vi "Check results (all plots).vi"(8 "error in":errorcluster, 9 "App Data":T1, 10 "XY Graph":refnum<vi>, 11 "ComboBox in":refnum<vi>) -> (0 "error out":errorcluster, 2 "results (short)":string, 3 "detailed results":string)   [LabVIEW 2014]
uses:
  Controls/App Data.ctl
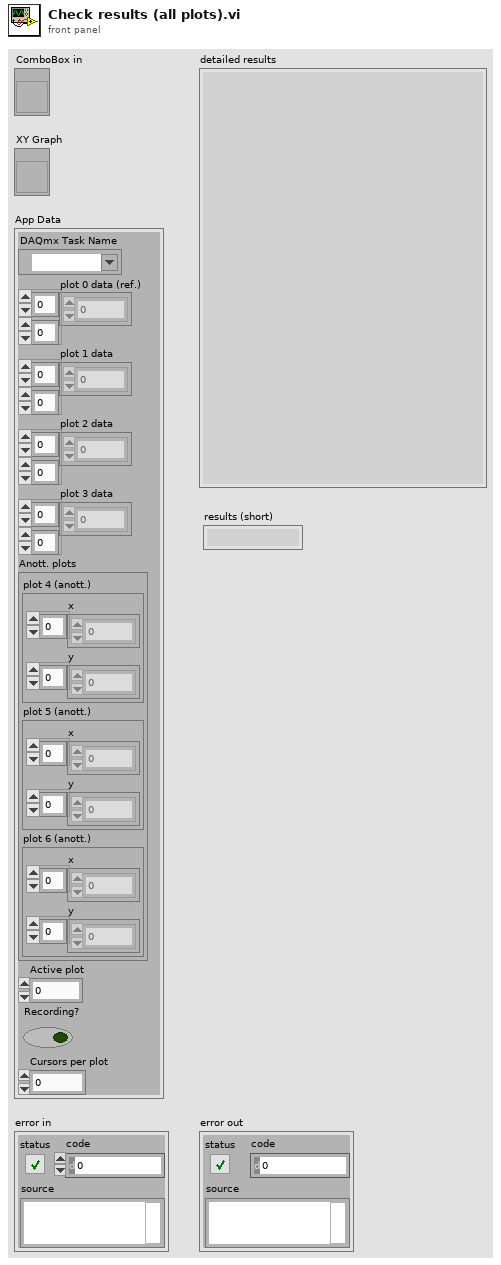
[diagram p1: front panel]
types:
  T1 = typedef "App Data.ctl" = cluster{"DAQmx Task Name":refnum<k21>, "plot 0 data (ref.)":dbl[][], "plot 1 data":dbl[][], "plot 2 data":dbl[][], "plot 3 data":dbl[][], "Anott. plots":cluster{"plot 4 (anott.)":cluster{"x":dbl[], "y":dbl[]}, "plot 5 (anott.)":cluster{"x":dbl[], "y":dbl[]}, "plot 6 (anott.)":cluster{"x":dbl[], "y":dbl[]}}, "Active plot":u32, "Recording?":bool, "Cursors per plot":i32}
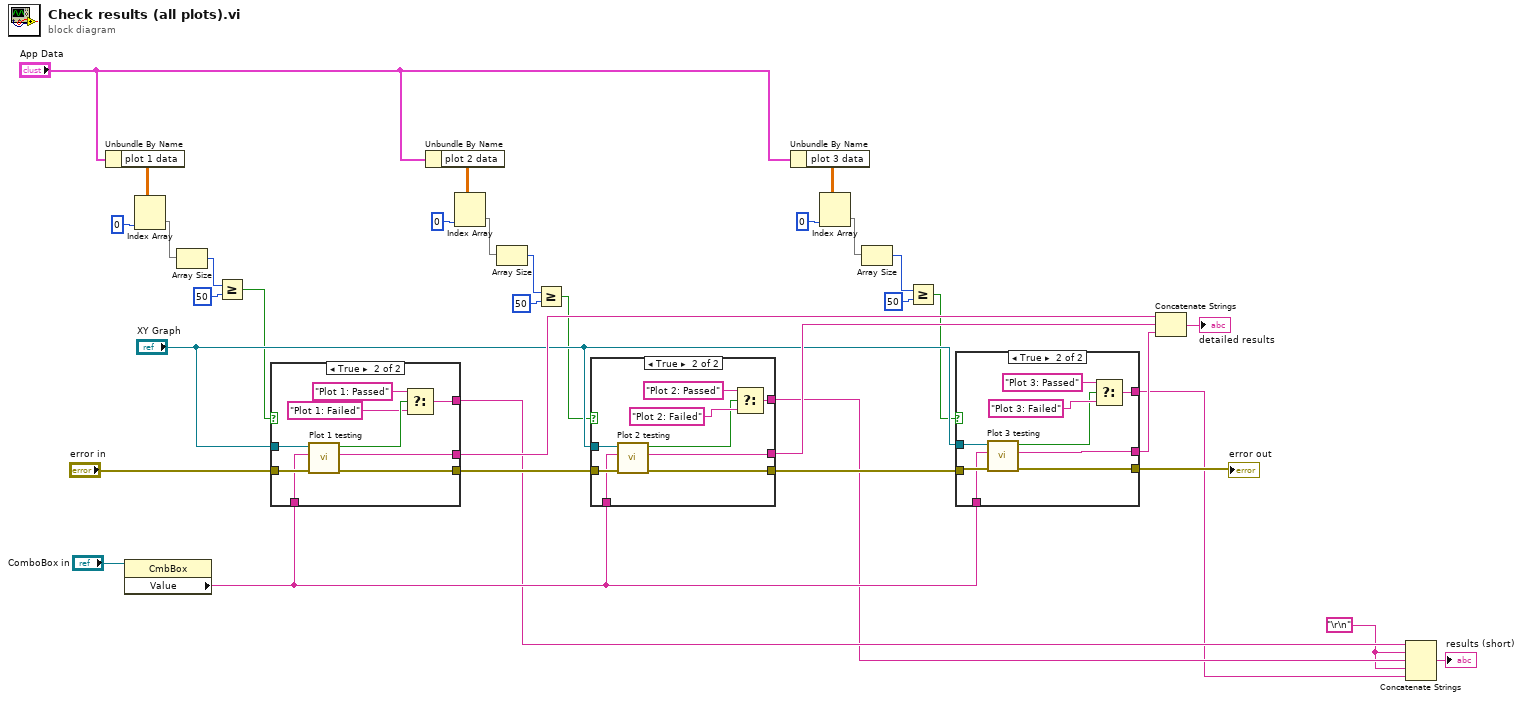
[diagram p0: block diagram]
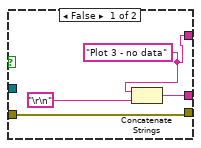
[diagram p2: hidden frame]
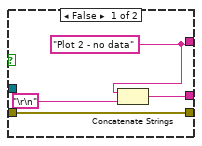
[diagram p3: hidden frame]
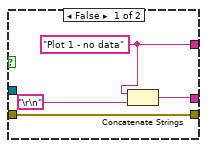
[diagram p4: hidden frame]
diagram:
  w3 = "\r\n"
  n1 = Unbundle By Name("App Data") -> ("plot 1 data"=w9:dbl[][])
  n2 = property class="CmbBox"(reference="ComboBox in") -> ("Value"=w31:string)  [unwired: 1 in, 2 out]
  n3 = Index Array(array=w9, index (col)=0 ("disabled index (col)")) -> (element=w10:dbl[])  [unwired: 1 in]
  n4 = Array Size(array=w10) -> (size(s)=w11:i32)
  n5 = Greater Or Equal?(x=w11, y=50) -> (x >= y?=w13:bool)
  n6 = case shown="True" w13 {
    tunnel: "error in" -> [w39 w48]
    tunnel: [w39 w47] -> w27
    tunnel: "XY Graph" -> [_ w46]
    tunnel: w31 -> [_ w45]
    tunnel: [w38 w44] -> w32
    tunnel: [w36 w40] -> w5
    frame False {
      w36 = "Plot 1 - no data" ("concatenated string 6")
      n7 = Concatenate Strings(w36, "\r\n") -> (w38:string)
    }
    frame True {
      n8 = call "Plot 1 testing.vi"("error in"=w48, "TWT type"=w45, "XY Graph"=w46) -> ("error out"=w47:errorcluster, "Results"=w44:string, "Plot 1 pass?"=w43:bool)  [unwired: 6 in]
      n9 = Select(t="Plot 1: Passed", s=w43, f="Plot 1: Failed") -> (s? t:f=w40:string)
    }
  }
  n10 = Unbundle By Name("App Data") -> ("plot 2 data"=w15:dbl[][])
  n11 = Index Array(array=w15, index (col)=0 ("disabled index (col)")) -> (element=w16:dbl[])  [unwired: 1 in]
  n12 = Array Size(array=w16) -> (size(s)=w17:i32)
  n13 = Greater Or Equal?(x=w17, y=50) -> (x >= y?=w19:bool)
  n14 = case shown="True" w19 {
    tunnel: w27 -> [w52 w61]
    tunnel: [w52 w60] -> w28
    tunnel: "XY Graph" -> [_ w59]
    tunnel: w31 -> [_ w58]
    tunnel: [w50 w57] -> w33
    tunnel: [w49 w53] -> w4
    frame False {
      w49 = "Plot 2 - no data" ("concatenated string 6")
      n15 = Concatenate Strings(w49, "\r\n") -> (w50:string)
    }
    frame True {
      n16 = call "Plot 2 testing.vi"("error in"=w61, "TWT type"=w58, "XY Graph"=w59) -> ("error out"=w60:errorcluster, "concatenated string 6"=w57:string, "Plot 2 pass?"=w54:bool)  [unwired: 6 in]
      n17 = Select(t="Plot 2: Passed", s=w54, f="Plot 2: Failed") -> (s? t:f=w53:string)
    }
  }
  n18 = Unbundle By Name("App Data") -> ("plot 3 data"=w21:dbl[][])
  n19 = Index Array(array=w21, index (col)=0 ("disabled index (col)")) -> (element=w22:dbl[])  [unwired: 1 in]
  n20 = Array Size(array=w22) -> (size(s)=w23:i32)
  n21 = Greater Or Equal?(x=w23, y=50) -> (x >= y?=w25:bool)
  n22 = case shown="True" w25 {
    tunnel: w28 -> [w65 w74]
    tunnel: [w65 w73] -> w29
    tunnel: "XY Graph" -> [_ w72]
    tunnel: w31 -> [_ w71]
    tunnel: [w63 w70] -> w34
    tunnel: [w62 w67] -> w2
    frame False {
      w62 = "Plot 3 - no data" ("concatenated string 6")
      n23 = Concatenate Strings(w62, "\r\n") -> (w63:string)
    }
    frame True {
      n24 = call "Plot 3 testing.vi"("error in"=w74, "TWT type"=w71, "XY Graph"=w72) -> ("error out"=w73:errorcluster, "concatenated string 6"=w70:string, "Plot 3 pass?"=w66:bool)  [unwired: 6 in]
      n25 = Select(t="Plot 3: Passed", s=w66, f="Plot 3: Failed") -> (s? t:f=w67:string)
    }
  }
  "error out" <- w29
  n26 = Concatenate Strings(w32, w33, w34) -> (→"detailed results":string)
  n27 = Concatenate Strings(w5, w3, w4, w3, w2) -> (→"results (short)":string)
